vi "Number to Time String.vi"(11 "Numeric":i32) -> (3 "String":string)   [LabVIEW 2013]
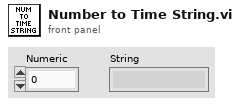
[diagram p1: front panel]
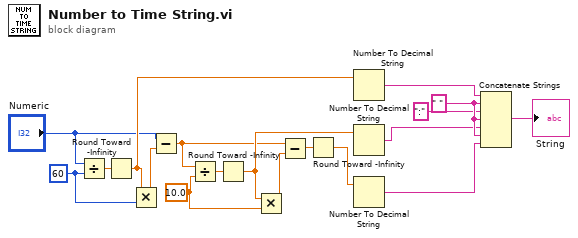
[diagram p0: block diagram]
diagram:
  w8 = " "
  w15 = 10.0 ("y")
  w13 = 60 ("y")
  n1 = Divide(x="Numeric", y=w13) -> (x/y=w11:dbl)
  n2 = Round Toward -Infinity(1:w11) -> (0:w17:dbl)
  n3 = Multiply(x=w17, y=w13) -> (x*y=w12:dbl)
  n4 = Subtract(x="Numeric", y=w12) -> (x-y=w2:dbl)
  n5 = Divide(x=w2, y=w15) -> (x/y=w14:dbl)
  n6 = Round Toward -Infinity(1:w14) -> (0:w18:dbl)
  n7 = Multiply(x=w18, y=w15) -> (x*y=w16:dbl)
  n8 = Subtract(x=w2, y=w16) -> (x-y=w3:dbl)
  n9 = Round Toward -Infinity(1:w3) -> (0:w4:dbl)
  n10 = Number To Decimal String(number=w17) -> (decimal integer string=w5:string)  [unwired: 1 in]
  n11 = Number To Decimal String(number=w18) -> (decimal integer string=w7:string)  [unwired: 1 in]
  n12 = Number To Decimal String(number=w4) -> (decimal integer string=w9:string)  [unwired: 1 in]
  n13 = Concatenate Strings(w5, w8, ":" ("string"), w8, w7, w8, w9) -> (→"String":string)
